vi "goal_with_force_Msg.vi"(8 "error in (no error)":errorcluster caption="错误输入（无错误）", 10 "值(信号)":T1, 11 "States.lvlib:Guide.lvclass":refnum<class "Guide.lvclass">) -> (0 "error out":errorcluster caption="错误输出", 3 "Process State out":refnum<class "State Actor.lvclass">)   [LabVIEW 2014, in "States.lvlib" / "Guide.lvclass"]
uses:
  Guide.lvclass
  <vilib>/NI/Actors/State Actor/State Actor/State Actor.lvclass
  <vilib>/ActorFramework/Message Enqueuer/Message Enqueuer.lvclass/Message Enqueuer.ctl
  <vilib>/ActorFramework/Message Enqueuer/Enqueue.vi
  <vilib>/ActorFramework/Message Priority Queue/Priority Enqueue.vi
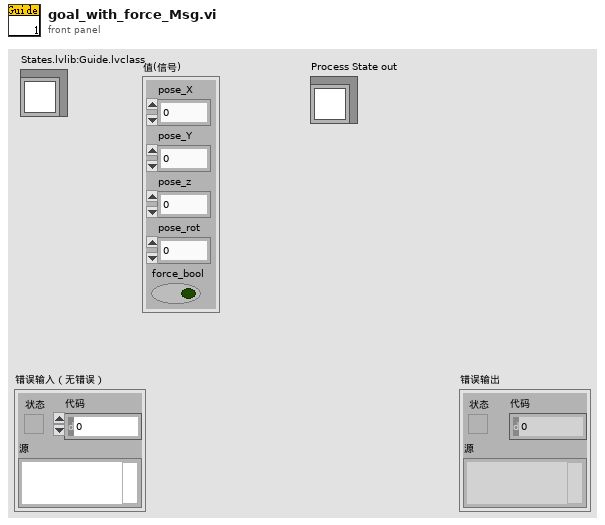
[diagram p1: front panel]
types:
  T1 = cluster{"pose_X":dbl, "pose_Y":dbl, "pose_z":dbl, "pose_rot":dbl, "force_bool":bool}
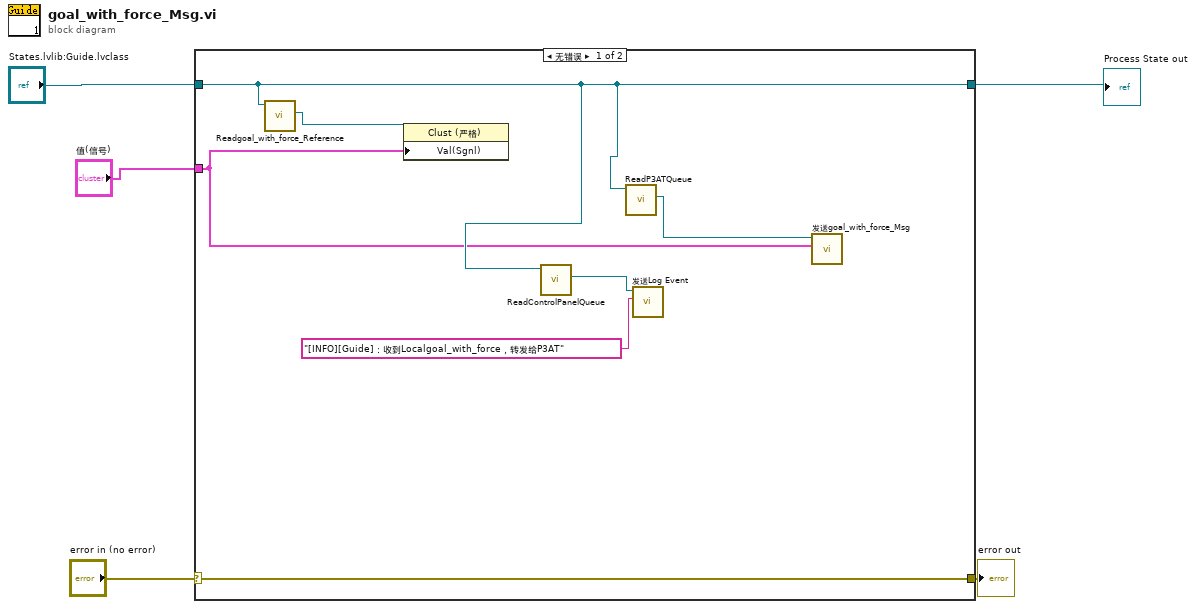
[diagram p0: block diagram]
diagram:
  n1 = case shown="无错误" "error in (no error)" {
    selector: "error in (no error)" -> [w12 w13]
    tunnel: [w12 w13] -> w4
    tunnel: [w9 w14] -> w3
    tunnel: "States.lvlib:Guide.lvclass" -> [w9 w14]
    tunnel: "值(信号)" -> [w6 _]
    frame No Error {
      n2 = call-dynamic "Readgoal_with_force_Reference.vi"("CoordinatorState输入"=w9) -> ("goal_with_force_Reference"=w11:refnum<vi>)  [unwired: 8 in, 2 out]
      n3 = property class="Clust (严格)"(reference=w11, "Val(Sgnl)"=w6) -> ()  [unwired: 1 in, 2 out]
      n4 = call-dynamic "ReadControlPanelQueue.vi"("CoordinatorState输入"=w9) -> ("操作者框架:消息待入队列"=w10:refnum<class "Message Enqueuer.lvclass">)  [unwired: 8 in, 2 out]
      n5 = call-dynamic "ReadP3ATQueue.vi"("CoordinatorState输入"=w9) -> ("操作者框架:消息待入队列"=w7:refnum<class "Message Enqueuer.lvclass">)  [unwired: 8 in, 2 out]
      n6 = call "发送Log Event.vi"("Event Text"="[INFO][Guide]：收到Localgoal_with_force，转发给P3AT", "消息待入队列"=w10) -> ()  [unwired: 8 in, 2 out]
      n7 = call "发送goal_with_force_Msg.vi"("值(信号)"=w6, "消息待入队列"=w7) -> ()  [unwired: 8 in, 2 out]
    }
    frame Error {
    }
  }
  "error out" <- w4
  "Process State out" <- w3
